vi "校准记录.vi"(8 "error in (no error)":errorcluster, 9 "曲线模型":T1={"标液浓度1"=0.0, "测量吸光度1"=0.0, "样品1启用"=FALSE, "标液浓度2"=0.0, "测量吸光度2"=0.0, "样品2启用"=FALSE, "标液浓度3"=0.0, "测量吸光度3"=0.0, "样品3启用"=FALSE, "标液浓度4"=0.0, "测量吸光度4"=0.0, "样品4启用"=FALSE, "标液浓度5"=0.0, "测量吸光度5"=0.0, "样品5启用"=FALSE, "模型"=enum."线性", "精度"=4.0, "XY图"=[], "拟合公式"="", "r^2"=0.0, "标样一校准时间"=timestamp(0 s since 1904-01-01), "标样二校准时间"=timestamp(0 s since 1904-01-01), "标样三校准时间"=timestamp(0 s since 1904-01-01), "标样四校准时间"=timestamp(0 s since 1904-01-01), "标样五校准时间"=timestamp(0 s since 1904-01-01), "二次方程"={"c"=0.0, "x"=0.0, "x^2"=0.0}, "标定时间"=timestamp(0 s since 1904-01-01), "拟合公式 2"="", "r^2 2"=0.0} {"r^2 2" format="%.7f"; "标定时间" format="%<%m/%d/%y %H:%M:%S>T"; "标样五校准时间" format="%<%m/%d/%y %H:%M:%S>T"; "标样四校准时间" format="%<%m/%d/%y %H:%M:%S>T"; "标样三校准时间" format="%<%m/%d/%y %H:%M:%S>T"; "标样二校准时间" format="%<%m/%d/%y %H:%M:%S>T"; "标样一校准时间" format="%<%m/%d/%y %H:%M:%S>T"; "r^2" format="%.7f"; "测量吸光度5" format="%#.6f"; "测量吸光度4" format="%#.6f"; "测量吸光度3" format="%#.6f"; "测量吸光度2" format="%#.6f"; "测量吸光度1" format="%#.6f"}, 10 "量程":enum16{"低量程", "高量程"}(ring), 11 "测量模式":string="所有测量模式") -> (0 "error out":errorcluster)   [LabVIEW 2016, in "斯坦道CODMn.lvlib"]
panel:
  out "结果字符串":string
  in  "data in":T2
  # "校准时间"
  # "标液浓度"
  # "吸光值显示"
  # "标液一"
  # "标液二"
  # "标液三"
  # "零点"
  # "跨度"
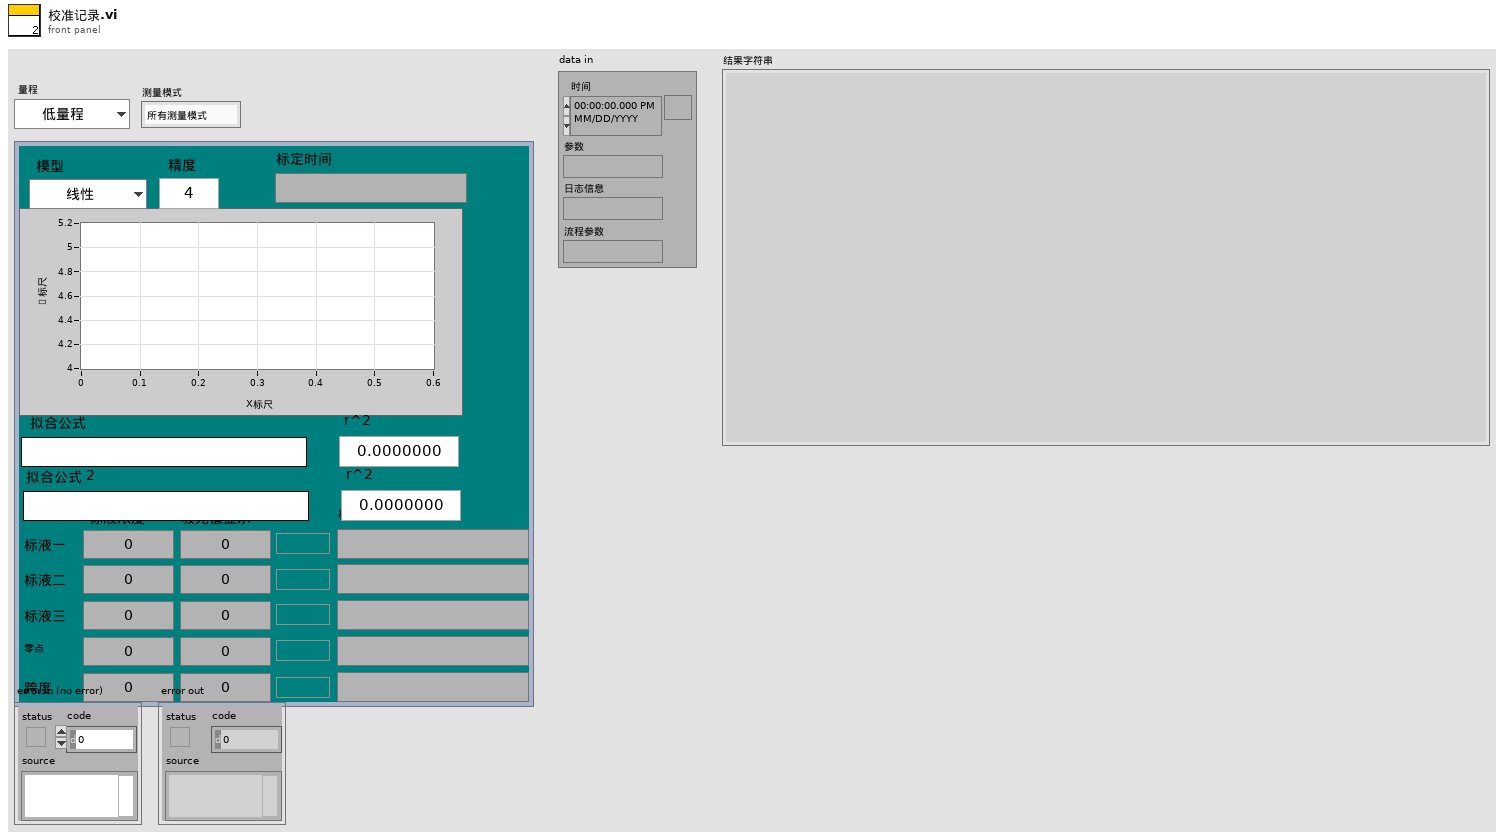
[diagram p1: front panel]
types:
  T1 = cluster{"标液浓度1":dbl, "测量吸光度1":dbl, "样品1启用":bool, "标液浓度2":dbl, "测量吸光度2":dbl, "样品2启用":bool, "标液浓度3":dbl, "测量吸光度3":dbl, "样品3启用":bool, "标液浓度4":dbl, "测量吸光度4":dbl, "样品4启用":bool, "标液浓度5":dbl, "测量吸光度5":dbl, "样品5启用":bool, "模型":enum32{"线性", "多项式", "折线"}, "精度":dbl, "XY图":cluster{"X Values":dbl[], "Y Values":dbl[]}[], "拟合公式":string, "r^2":dbl, "标样一校准时间":timestamp, "标样二校准时间":timestamp, "标样三校准时间":timestamp, "标样四校准时间":timestamp, "标样五校准时间":timestamp, "二次方程":cluster{"c":dbl, "x":dbl, "x^2":dbl}, "标定时间":timestamp, "拟合公式 2":string, "r^2 2":dbl}
  T2 = cluster{"时间":timestamp, "参数":string, "日志信息":string, "流程参数":string}
  T3 = cluster{"低标液1浓度":dbl, "低标液1信号值":dbl, "低标液1启用":u16, "低标液2浓度":dbl, "低标液2信号值":dbl, "低标液2启用":u16, "低标液3浓度":dbl, "低标液3信号值":dbl, "低标液3启用":u16, "低标液4浓度":dbl, "低标液4信号值":dbl, "低标液4启用":u16, "低标液5浓度":dbl, "低标液5信号值":dbl, "低标液5启用":u16, "高标液1浓度":dbl, "高标液1信号值":dbl, "高标液1启用":u16, "高标液2浓度":dbl, "高标液2信号值":dbl, "高标液2启用":u16, "高标液3浓度":dbl, "高标液3信号值":dbl, "高标液3启用":u16, "高标液4浓度":dbl, "高标液4信号值":dbl, "高标液4启用":u16, "高标液5浓度":dbl, "高标液5信号值":dbl, "高标液5启用":u16}
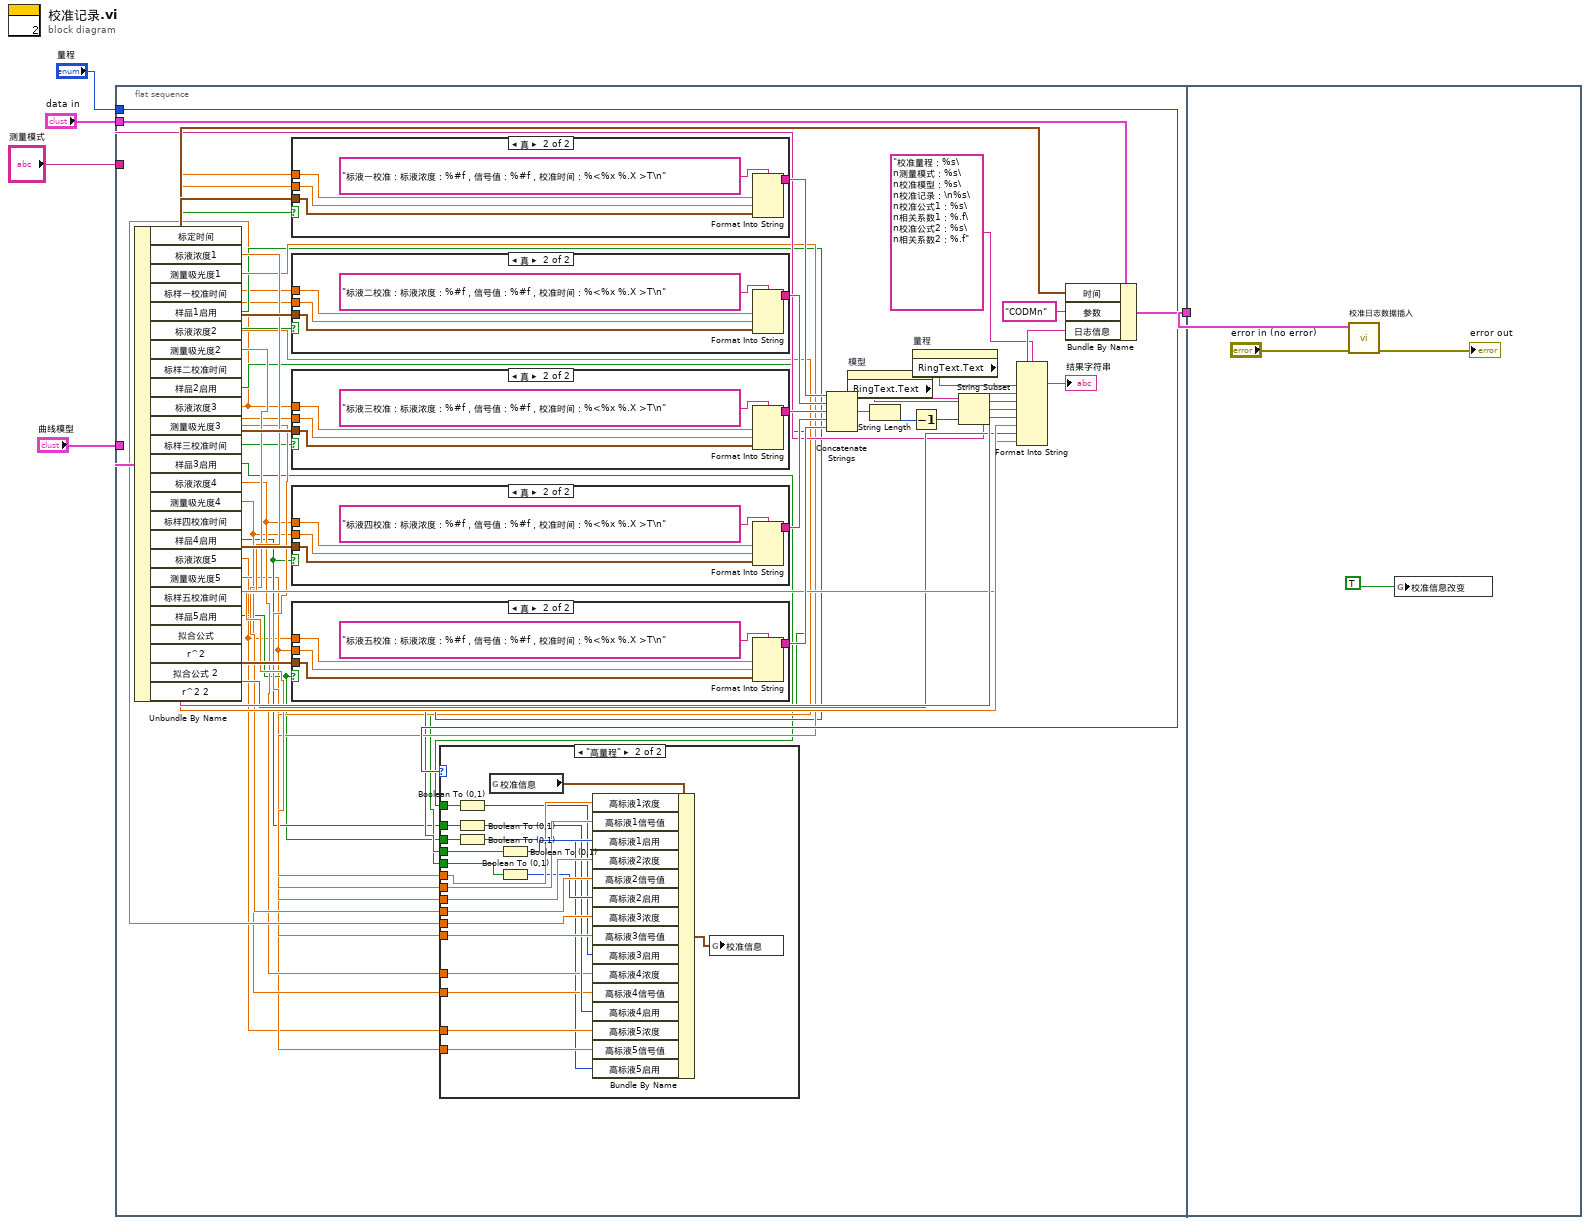
[diagram p0: block diagram]
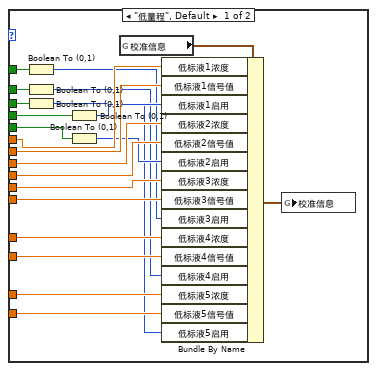
[diagram p2: hidden frame]
diagram:
  n1 = flat-sequence {
    tunnel: "量程" -> [w21]
    tunnel: "曲线模型" -> [w45]
    tunnel: "data in" -> [w49]
    tunnel: [w48] -> w2
    tunnel: "测量模式" -> [w22]
    tunnel: w2 -> [w120]
    frame #0 {
      n2 = Unbundle By Name(w45) -> ("标定时间"=w28:timestamp, "标液浓度1"=w20:dbl, "测量吸光度1"=w19:dbl, "标样一校准时间"=w44:timestamp, "样品1启用"=w18:bool, "标液浓度2"=w17:dbl, "测量吸光度2"=w16:dbl, "标样二校准时间"=w43:timestamp, "样品2启用"=w15:bool, "标液浓度3"=w14:dbl, "测量吸光度3"=w13:dbl, "标样三校准时间"=w42:timestamp, "样品3启用"=w12:bool, "标液浓度4"=w11:dbl, "测量吸光度4"=w10:dbl, "标样四校准时间"=w41:timestamp, "样品4启用"=w9:bool, "标液浓度5"=w6:dbl, "测量吸光度5"=w7:dbl, "标样五校准时间"=w40:timestamp, "样品5启用"=w8:bool, "拟合公式"=w34:string, "r^2"=w33:dbl, "拟合公式 2"=w26:string, "r^2 2"=w27:dbl)
      n3 = case shown="真" w18 {
        tunnel: w20 -> [_ w117]
        tunnel: w19 -> [_ w116]
        tunnel: w44 -> [_ w115]
        tunnel: [_ w114] -> w39
        frame False {
        }
        frame True {
          n4 = Format Into String(format string="标液一校准：标液浓度：%#f，信号值：%#f，校准时间：%<%x %.X >T\n" ("格式字符串"), w117, w116, w115) -> (resulting string=w114:string)  [unwired: 2 in, 1 out]
        }
      }
      n5 = case shown="真" w15 {
        tunnel: w17 -> [_ w112]
        tunnel: w16 -> [_ w111]
        tunnel: w43 -> [_ w110]
        tunnel: [_ w109] -> w38
        frame False {
        }
        frame True {
          n6 = Format Into String(format string="标液二校准：标液浓度：%#f，信号值：%#f，校准时间：%<%x %.X >T\n" ("格式字符串"), w112, w111, w110) -> (resulting string=w109:string)  [unwired: 2 in, 1 out]
        }
      }
      n7 = case shown="真" w12 {
        tunnel: w14 -> [_ w107]
        tunnel: w13 -> [_ w106]
        tunnel: w42 -> [_ w105]
        tunnel: [_ w104] -> w37
        frame False {
        }
        frame True {
          n8 = Format Into String(format string="标液三校准：标液浓度：%#f，信号值：%#f，校准时间：%<%x %.X >T\n" ("格式字符串"), w107, w106, w105) -> (resulting string=w104:string)  [unwired: 2 in, 1 out]
        }
      }
      n9 = case shown="真" w9 {
        tunnel: w11 -> [_ w102]
        tunnel: w10 -> [_ w101]
        tunnel: w41 -> [_ w100]
        tunnel: [_ w99] -> w36
        frame False {
        }
        frame True {
          n10 = Format Into String(format string="标液四校准：标液浓度：%#f，信号值：%#f，校准时间：%<%x %.X >T\n" ("格式字符串"), w102, w101, w100) -> (resulting string=w99:string)  [unwired: 2 in, 1 out]
        }
      }
      n11 = case shown="真" w8 {
        tunnel: w6 -> [_ w97]
        tunnel: w7 -> [_ w96]
        tunnel: w40 -> [_ w95]
        tunnel: [_ w94] -> w35
        frame False {
        }
        frame True {
          n12 = Format Into String(format string="标液五校准：标液浓度：%#f，信号值：%#f，校准时间：%<%x %.X >T\n" ("格式字符串"), w97, w96, w95) -> (resulting string=w94:string)  [unwired: 2 in, 1 out]
        }
      }
      n13 = case shown="\"高量程\"" w21 {
        tunnel: w20 -> [w71 w91]
        tunnel: w19 -> [w70 w90]
        tunnel: w18 -> [w68 w93]
        tunnel: w17 -> [w69 w89]
        tunnel: w16 -> [w66 w88]
        tunnel: w15 -> [w65 w87]
        tunnel: w14 -> [w63 w85]
        tunnel: w13 -> [w62 w84]
        tunnel: w12 -> [w61 w83]
        tunnel: w11 -> [w59 w78]
        tunnel: w10 -> [w58 w79]
        tunnel: w9 -> [w57 w81]
        tunnel: w8 -> [w52 w77]
        tunnel: w7 -> [w54 w75]
        tunnel: w6 -> [w55 w76]
        frame "低量程", Default {
          n14 = Boolean To (0,1)(Boolean=w61) -> (0, 1=w60:i16)
          n15 = Boolean To (0,1)(Boolean=w57) -> (0, 1=w56:i16)
          n16 = Boolean To (0,1)(Boolean=w52) -> (0, 1=w53:i16)
          n17 = Boolean To (0,1)(Boolean=w68) -> (0, 1=w67:i16)
          n18 = Boolean To (0,1)(Boolean=w65) -> (0, 1=w64:i16)
          n19 = global read "CODMn断电保存全局变量.vi" "校准信息"() -> (w50:T3)
          n20 = Bundle By Name(cluster=w50, "低标液1浓度"=w71, "低标液1信号值"=w70, "低标液1启用"=w67, "低标液2浓度"=w69, "低标液2信号值"=w66, "低标液2启用"=w64, "低标液3浓度"=w63, "低标液3信号值"=w62, "低标液3启用"=w60, "低标液4浓度"=w59, "低标液4信号值"=w58, "低标液4启用"=w56, "低标液5浓度"=w55, "低标液5信号值"=w54, "低标液5启用"=w53) -> (w51:T3)
          n21 = global write "CODMn断电保存全局变量.vi" "校准信息"(w51) -> ()
        }
        frame "高量程" {
          n22 = Boolean To (0,1)(Boolean=w83) -> (0, 1=w82:i16)
          n23 = Boolean To (0,1)(Boolean=w81) -> (0, 1=w80:i16)
          n24 = Boolean To (0,1)(Boolean=w77) -> (0, 1=w74:i16)
          n25 = global read "CODMn断电保存全局变量.vi" "校准信息"() -> (w72:T3)
          n26 = Boolean To (0,1)(Boolean=w93) -> (0, 1=w92:i16)
          n27 = Boolean To (0,1)(Boolean=w87) -> (0, 1=w86:i16)
          n28 = Bundle By Name(cluster=w72, "高标液1浓度"=w91, "高标液1信号值"=w90, "高标液1启用"=w92, "高标液2浓度"=w89, "高标液2信号值"=w88, "高标液2启用"=w86, "高标液3浓度"=w85, "高标液3信号值"=w84, "高标液3启用"=w82, "高标液4浓度"=w78, "高标液4信号值"=w79, "高标液4启用"=w80, "高标液5浓度"=w76, "高标液5信号值"=w75, "高标液5启用"=w74) -> (w73:T3)
          n29 = global write "CODMn断电保存全局变量.vi" "校准信息"(w73) -> ()
        }
      }
      n30 = Concatenate Strings(w39, w38, w37, w36, w35) -> (w31:string)
      n31 = property on="模型" class="Enum (严格)"() -> ("RingText.Text"=w25:string)  [unwired: 2 in, 2 out]
      n32 = String Length(string=w31) -> (length=w30:i32)
      n33 = Decrement(x=w30) -> (x-1=w29:i32)
      n34 = property on="量程" class="Enum (严格)"() -> ("RingText.Text"=w23:string)  [unwired: 2 in, 2 out]
      n35 = String Subset(string=w31, length (rest)=w29) -> (substring=w32:string)  [unwired: 1 in]
      n36 = Format Into String(format string="校准量程：%s\n测量模式：%s\n校准模型：%s\n校准记录：\n%s\n校准公式1：%s\n相关系数1：%.f\n校准公式2：%s\n相关系数2：%.f" ("格式字符串"), w23, w22, w25, w32, w34, w33, w26, w27) -> (resulting string=w47:string)  [unwired: 2 in, 1 out]
      "结果字符串" <- w47
      n37 = Bundle By Name(cluster=w49, "时间"=w28, "参数"="CODMn", "日志信息"=w47) -> (w48:T2)
    }
    frame #1 {
      n38 = call "校准日志数据插入.vi"("data"=w120, "错误输入（无错误）"="error in (no error)") -> ("错误输出"=→"error out":errorcluster)  [unwired: 8 in]
      n39 = global write "CODMn断电保存全局变量.vi" "校准信息改变"(TRUE ("关键参数改变")) -> ()
    }
  }
